vi "context add verify paths.vi"(8 "error in":errorcluster, 10 "file":string, 11 "connector":u64) -> (0 "error out":errorcluster)   [LabVIEW 2016, in "async tls.lvlib"]
uses:
  async tls.lvlib
  lvasynctls.dll
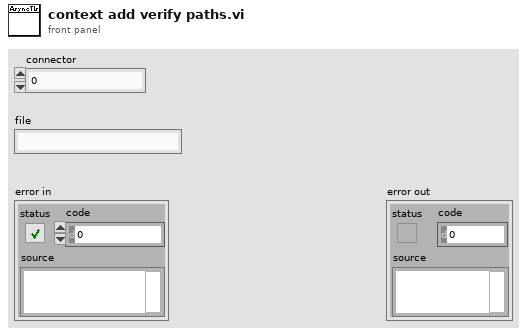
[diagram p1: front panel]
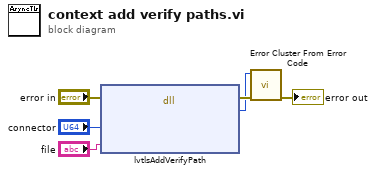
[diagram p0: block diagram]
diagram:
  n1 = dll-call lib="C:/Users/IEUser/Desktop/libasynclvtls/lvasynctls.dll" fn="lvtlsAddVerifyPath"(error in="error in", "connCreator"="connector", "file"="file") -> (error out=w6:errorcluster, "err"=w5:i32)  [unwired: 4 in, 1 out]
  n2 = call <vilib>:"Error Cluster From Error Code.vi"("error in (no error)"=w6, "error code (0)"=w5) -> ("error out"=→"error out":errorcluster)  [unwired: 7 in]
